vi "TLB Native Dynamic Events ver 0.04c.vi"() -> ()   [LabVIEW 2018]
uses:
  Labview Training Phase 2/Enum Controls/States for Action Engine.ctl
  Type def/TLB event states.ctl
  Type def/TLB MHL States.ctl
  <vilib>/Studica/Studica Toolkit/Background/I2C Channel.ctl
  <vilib>/Studica/Studica Toolkit/NavX/NavX.lvlib
  <vilib>/myRIO/Common/Instrument Driver Framework/myRIO v1.0/AI/typedefs/AI Channels Enum.ctl
  <vilib>/myRIO/Common/Instrument Driver Framework/myRIO v1.0/AI/typedefs/AI Channels List.ctl
  <vilib>/Studica/Studica Toolkit/Background/Mxp Selection.ctl
  <vilib>/ptbypt/NI_PtbyPt.lvlib
panel:
  out "Sharp IR Distance":dbl
  out "Sharp IR Distance 2":dbl
  out "CM":fxp<+,64,16>
  out "mean":dbl format="%0.2f"
  out "Waveform Chart 3":dbl(graph)
  out "NavX Info Out":T2
  out "LinearAcceleration":T3
  out "Displacement":T4
  out "YRPHfH":T5
  in  "xTargetSpeed":dbl
  in  "yTargetSpeed":dbl
  in  "wTargetSpeed":dbl
  out "Speed":T6
  in  "Reset Encoder 0":bool
  out "yDistance":dbl
  out "xDistance":dbl
  out "wDistance":dbl
  out "Action Queue Items":i32
  out "State Logic Queue Items":i32
  out "Action Queues items":string[](array[string])=["Hardware reset", "Software reset", ""]
  out "State logic":T7=enum."Task 2"
  out "Action State":string
  in  "Task Execution Mode":bool
  in  "Tasks Selector":string(combo)="Task 2"
  in  "Stop Queue":bool
  in  "Start Task":bool
  # "Test Programme written by Calvin Loke    Dated: 28 Aug 2019\nTest Programme revised by Dr Alex See   Dated 30 Aug 2019\n\nProgramme version:   TLB Native Dynamic Events ver 0.04b.vi"
  # "System Health Status Update"
  # "Sequence of Actions"
  # "Continuous (Repeated)"
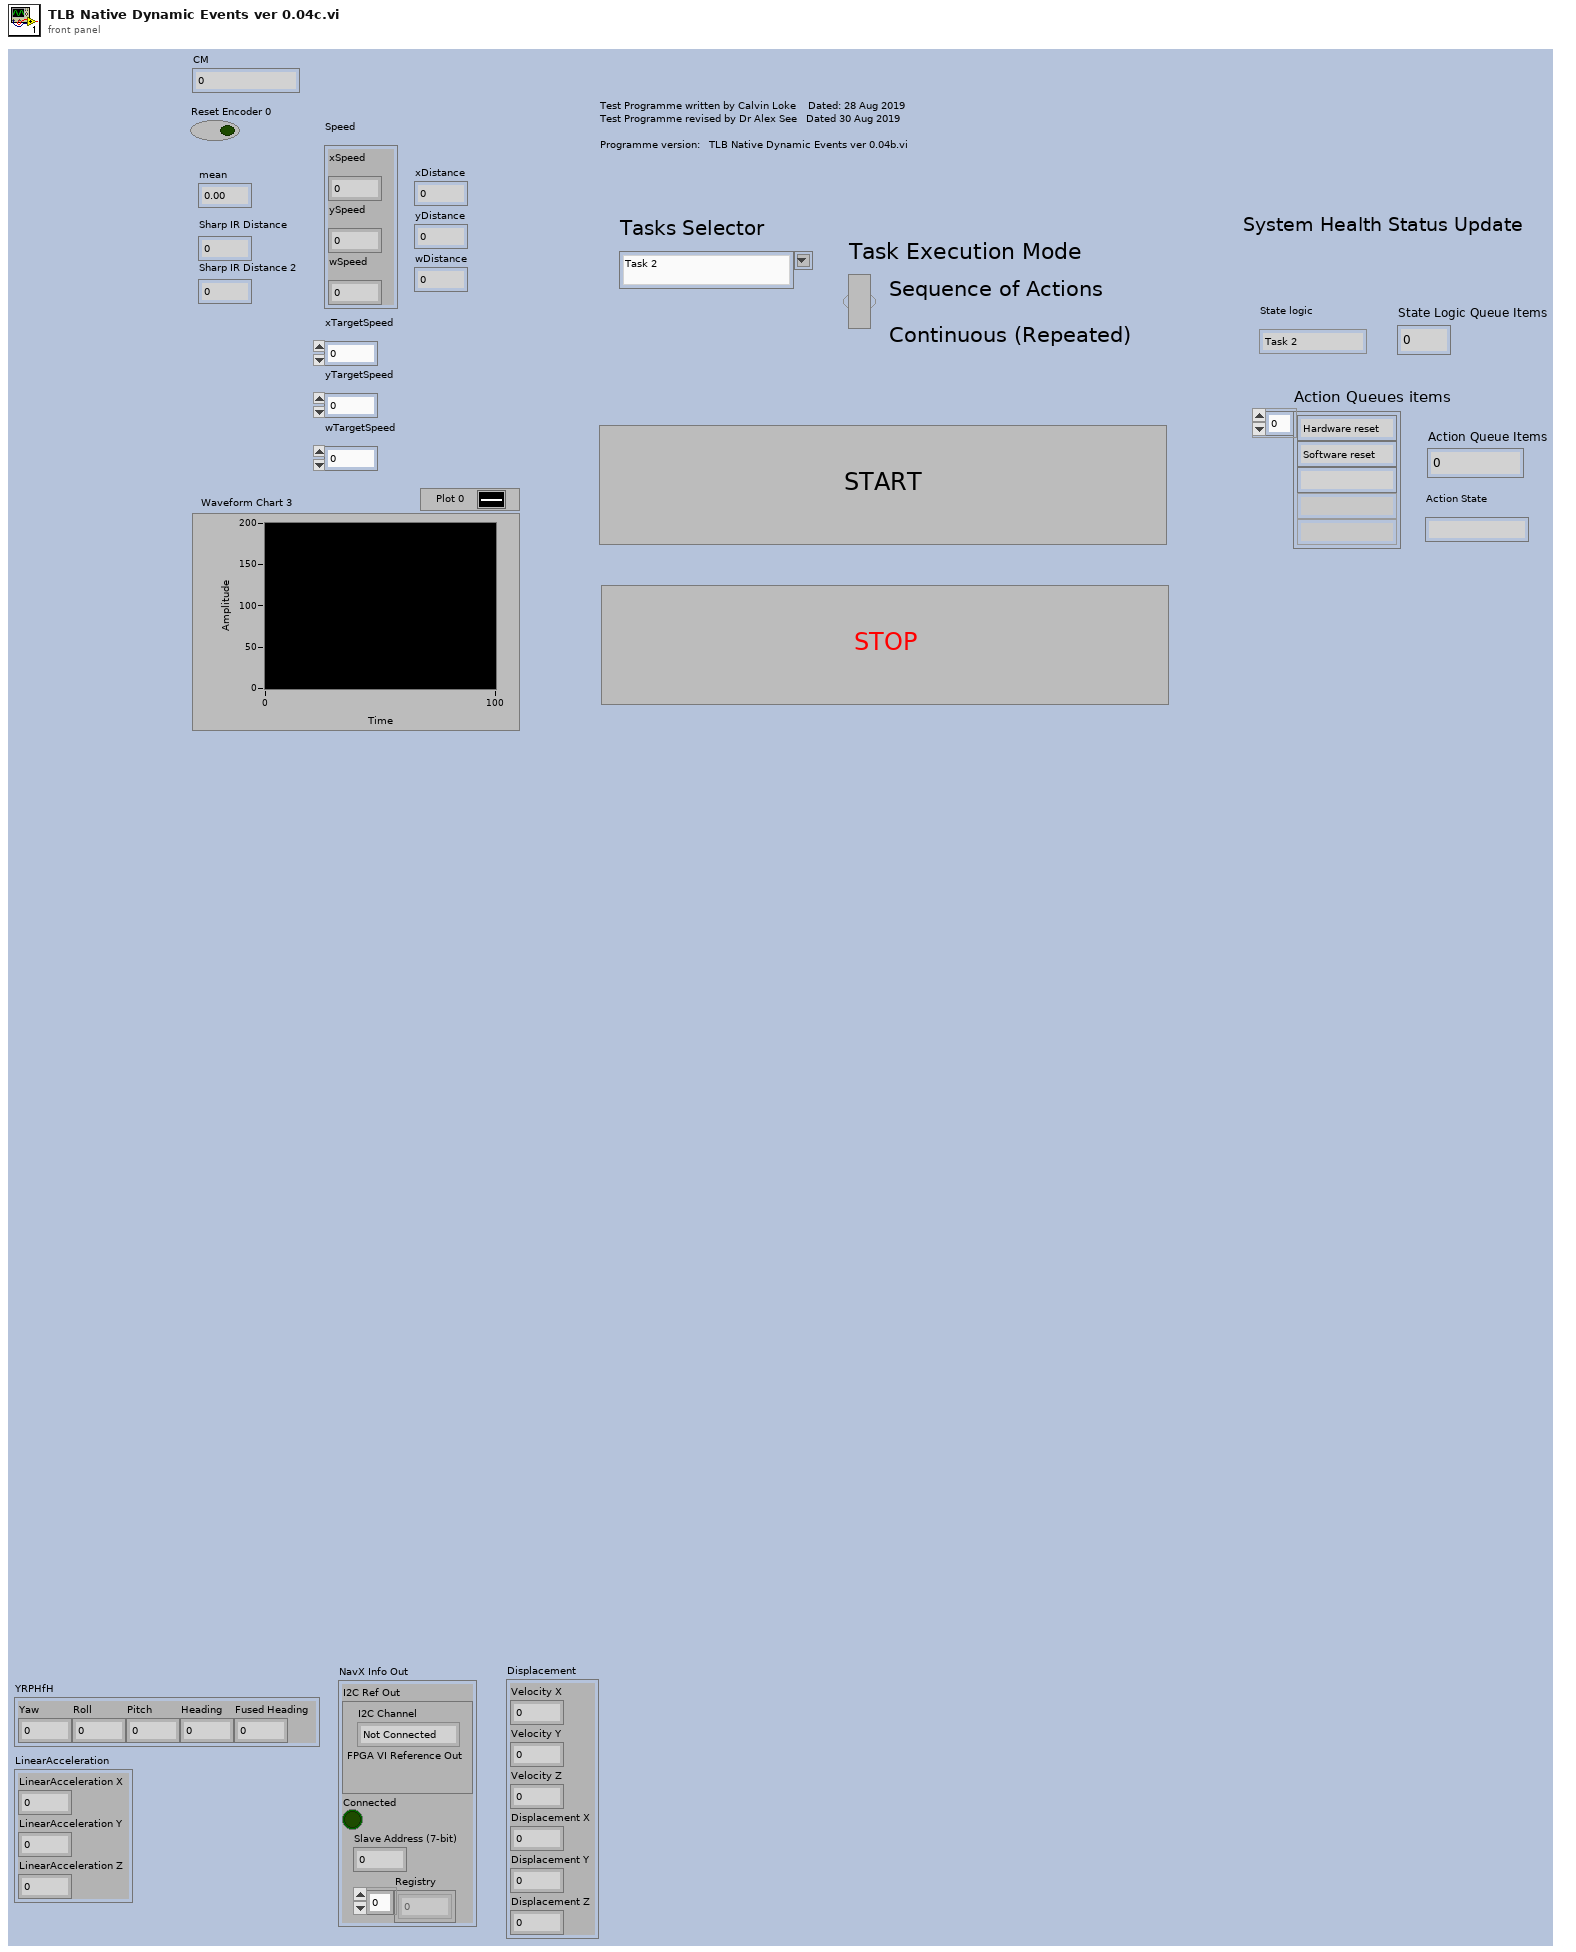
[diagram p1: front panel]
types:
  T1 = typedef "I2C Channel.ctl" = enum16{"Not Connected", "A", "B"}
  T2 = cluster{"I2C Ref Out":cluster{"I2C Channel":T1, "FPGA VI Reference Out":refnum<k20>}, "Connected":bool, "Slave Address (7-bit)":u8, "Registry":u8[]}
  T3 = cluster{"LinearAcceleration X":dbl, "LinearAcceleration Y":dbl, "LinearAcceleration Z":dbl}
  T4 = cluster{"Velocity X":dbl, "Velocity Y":dbl, "Velocity Z":dbl, "Displacement X":dbl, "Displacement Y":dbl, "Displacement Z":dbl}
  T5 = cluster{"Yaw":dbl, "Roll":dbl, "Pitch":dbl, "Heading":dbl, "Fused Heading":dbl}
  T6 = cluster{"xSpeed":dbl, "ySpeed":dbl, "wSpeed":dbl}
  T7 = typedef "TLB MHL States.ctl" = enum16{"None", "Startup", "Idle", "Processing", "Shutdown", "Reset", "Task 1", "Task 2", "Task 3", "Task 4", "Task 4a", "Task 4b", "Task 4c", "Task 4d", "Task 4e", "Task 4f", "Task 4g", "Task 4h", "Acquire image", "Wall follow mode", "Drive Straight"}
  T8 = typedef "States for Action Engine.ctl" = enum16{"Initialize", "Write", "Read"}
  T9 = typedef "TLB event states.ctl" = enum16{"Start Sequence", "Exit", "Start Task 1", "Start Task 2", "Start Task 3", "Start Task 4", "Camera vision", "Wall follow mode", "Idle", "Start Drive Straight"}
  T10 = typedef "Mxp Selection.ctl" = enum16{"MXP A", "MXP B"}
  T11 = typedef "TLB event states.ctl" = enum16{"Start Sequence", "Exit", "Task 1", "Task 2", "Idle"}
  T12 = typedef "AI Channels List.ctl" = T13[]
  T13 = typedef "AI Channels Enum.ctl" = enum16{"Not Connected", "AudioIn/Left", "AudioIn/Right", "C/AI0", "C/AI1", "A/AI0", "A/AI1", "A/AI2", "A/AI3", "A/AI4", "A/AI5", "A/AI6", "A/AI7", "B/AI0", "B/AI1", "B/AI2", "B/AI3", "B/AI4", "B/AI5", "B/AI6", "B/AI7", "AI/AI0", "AI/AI1", "AI/AI2", "AI/AI3", "A/AI0 (DIFF)", "A/AI1 (DIFF)", "A/AI2 (DIFF)", "A/AI3 (DIFF)", "B/AI0 (DIFF)", "B/AI1 (DIFF)", "B/AI2 (DIFF)", "B/AI3 (DIFF)"}
  T14 = cluster{"xDistance":dbl, "yDistance":dbl, "wDistance":dbl}
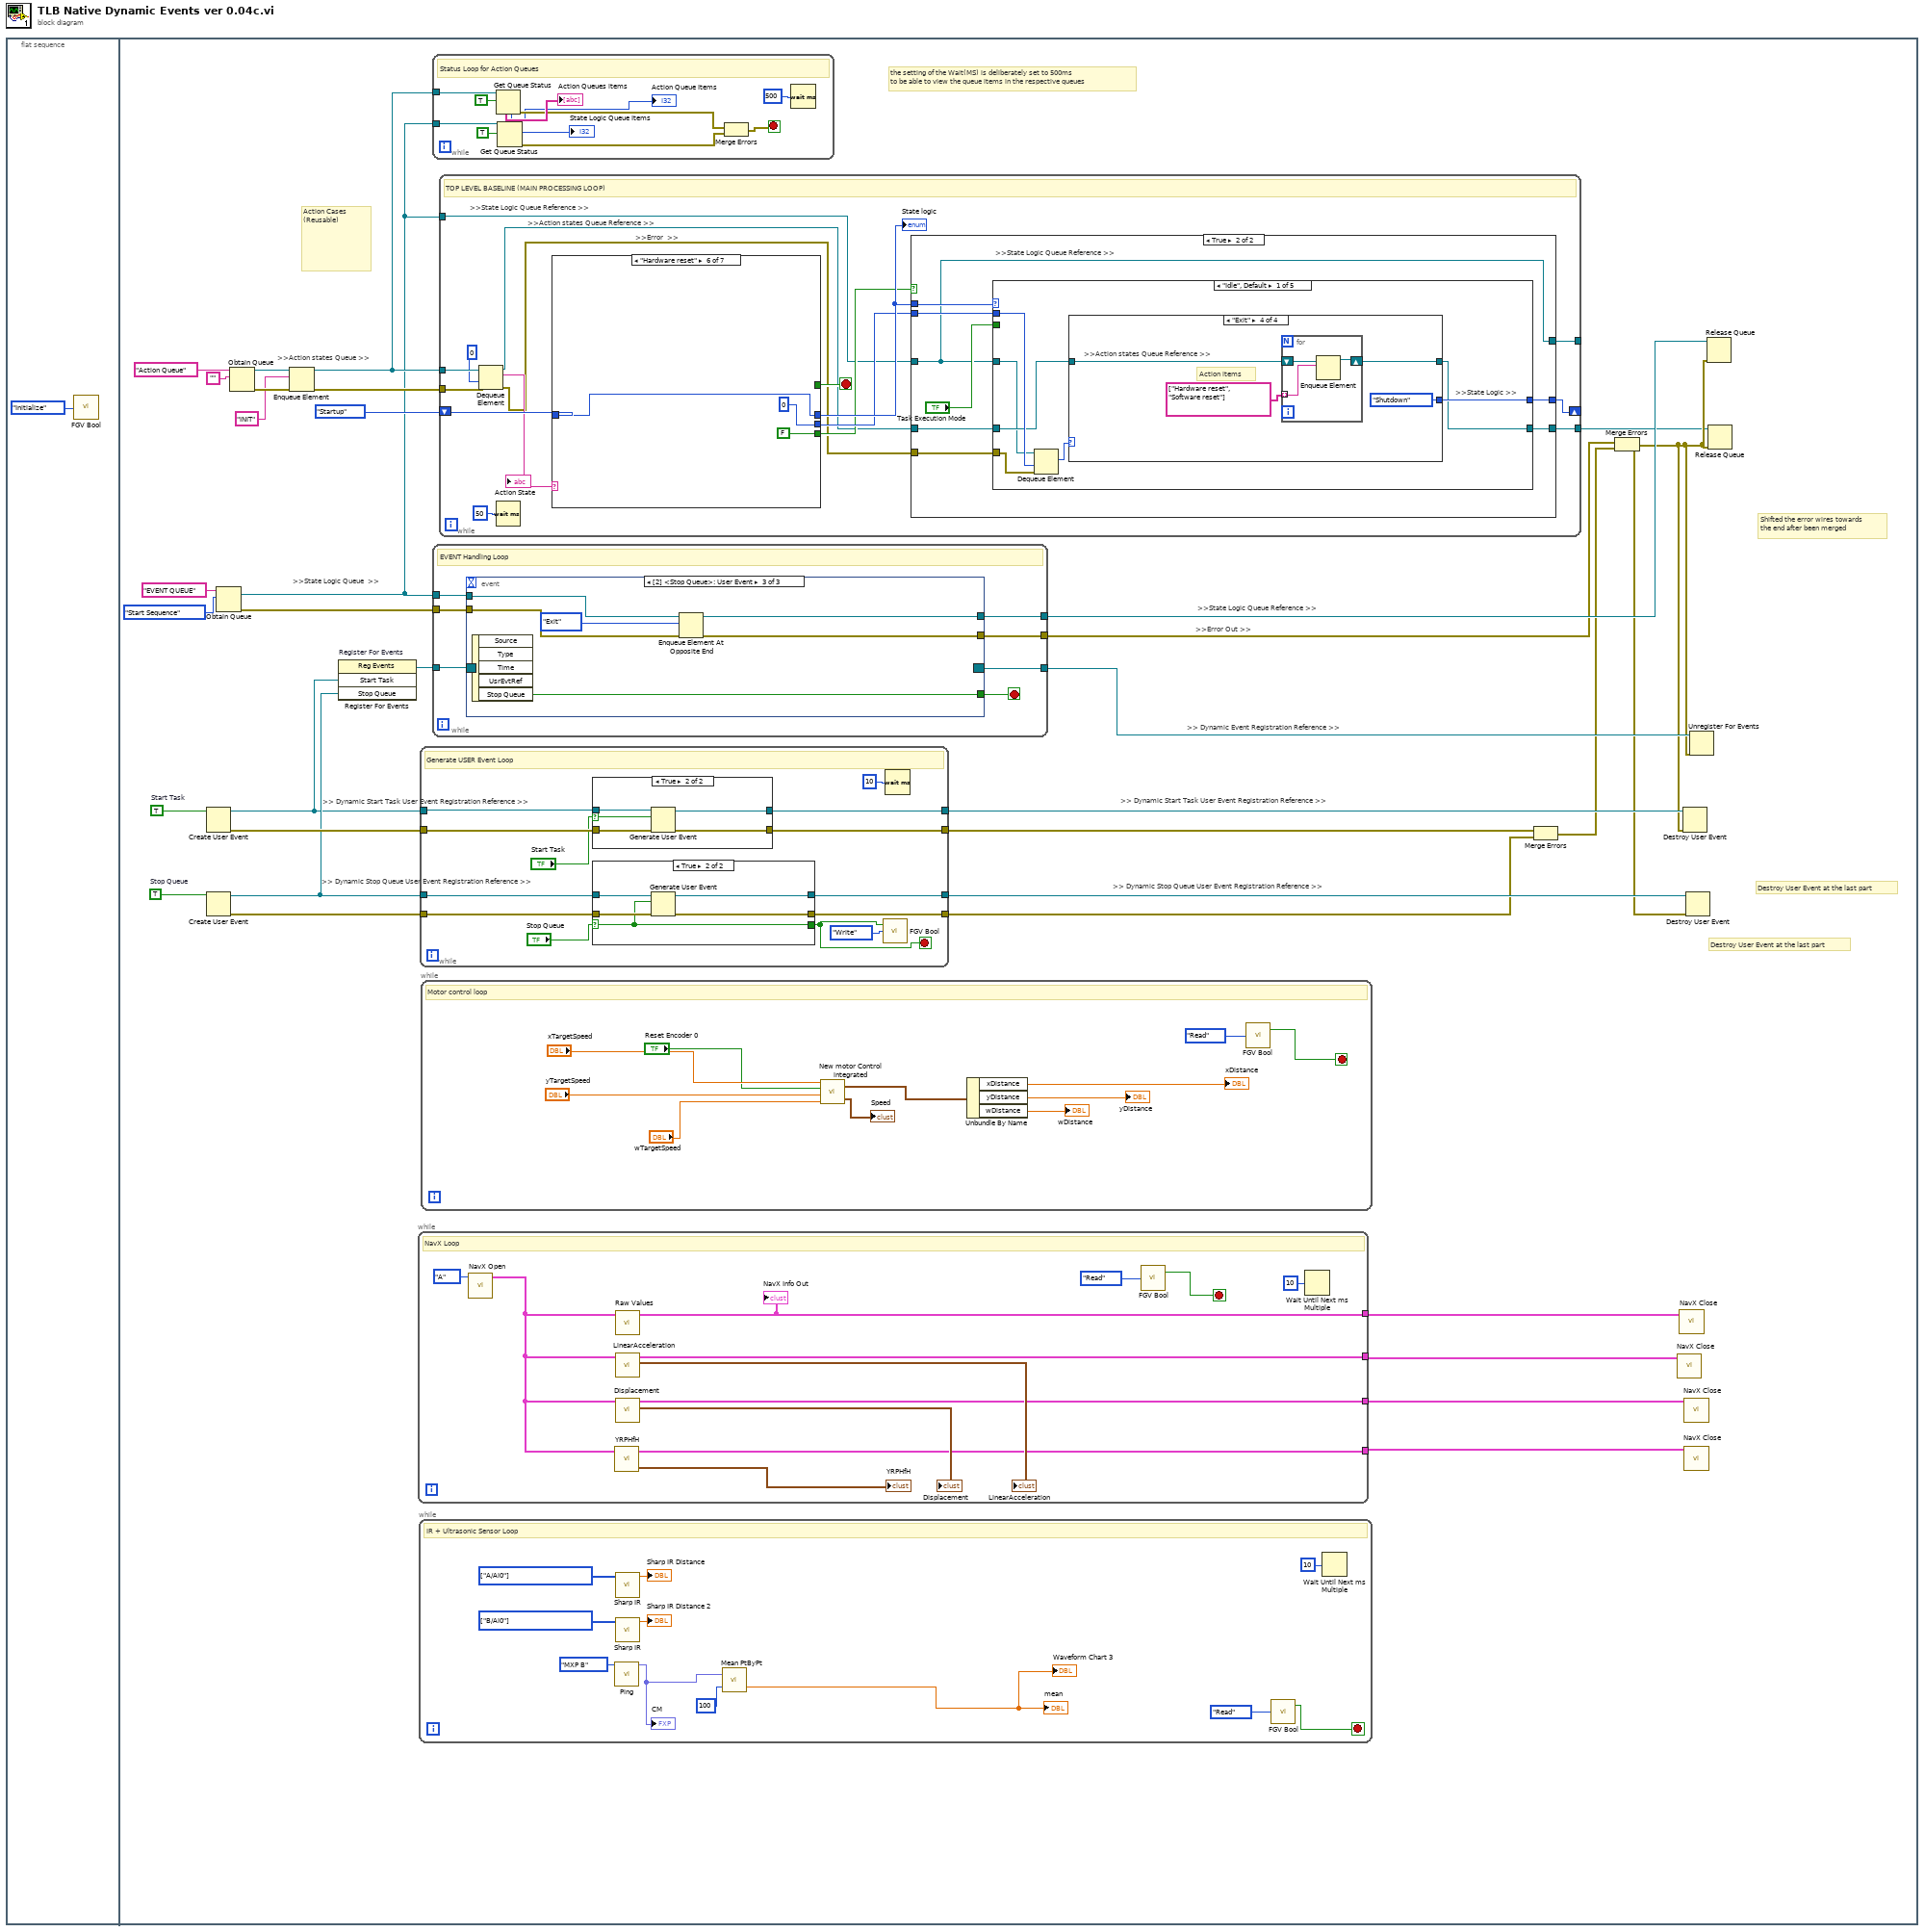
[diagram p0: block diagram]
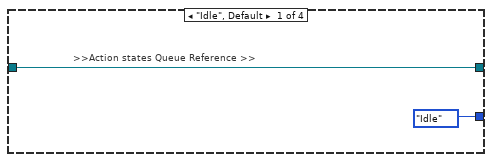
[diagram p3: hidden frame]
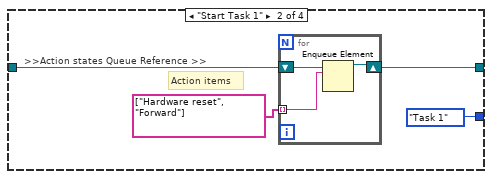
[diagram p4: hidden frame]
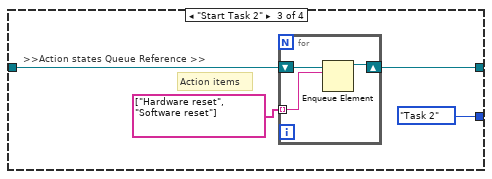
[diagram p5: hidden frame]
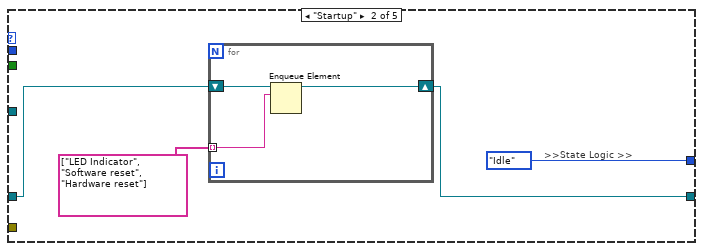
[diagram p6: hidden frame]
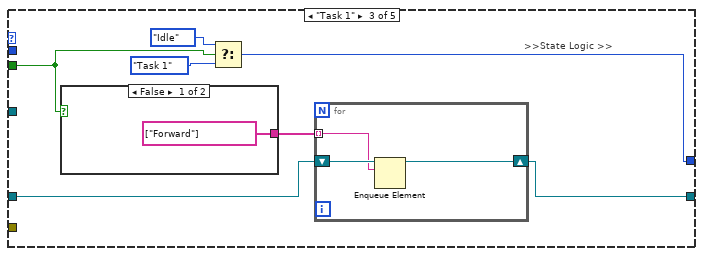
[diagram p7: hidden frame]
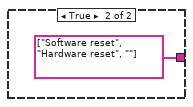
[diagram p8: hidden frame]
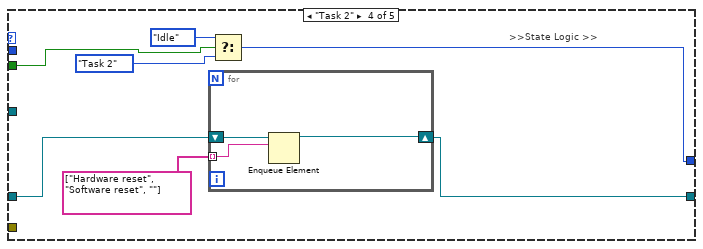
[diagram p9: hidden frame]
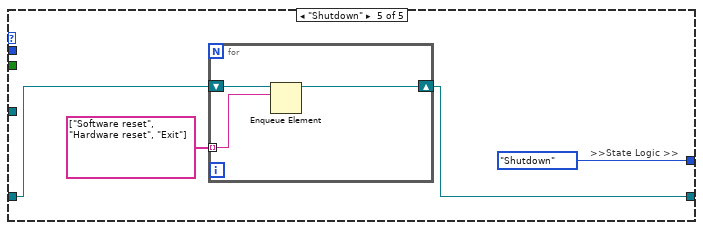
[diagram p10: hidden frame]
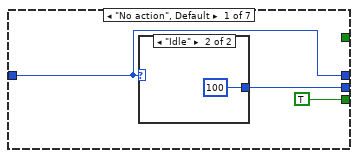
[diagram p11: hidden frame]
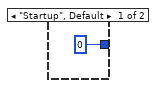
[diagram p12: hidden frame]
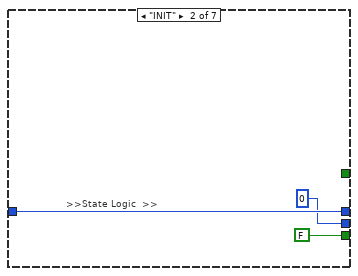
[diagram p13: hidden frame]
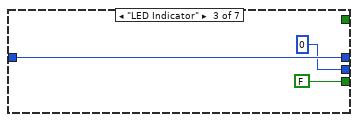
[diagram p14: hidden frame]
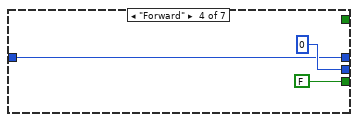
[diagram p15: hidden frame]
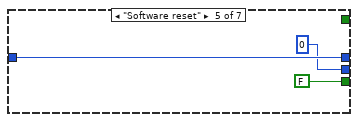
[diagram p16: hidden frame]
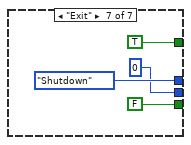
[diagram p17: hidden frame]
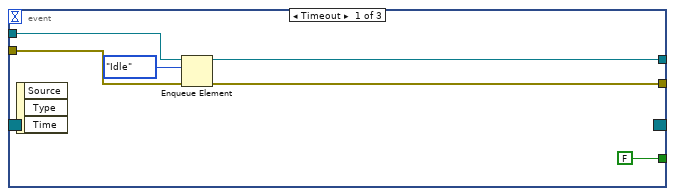
[diagram p18: hidden frame]
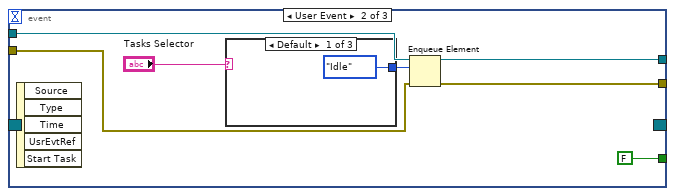
[diagram p19: hidden frame]
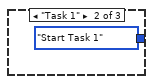
[diagram p20: hidden frame]
diagram:
  n1 = flat-sequence {
    frame #0 {
      n2 = call "FGV Bool.vi"("Init/Read/Write State"=States_for_Action_Engine."Initialize") -> ()  [unwired: 2 in, 2 out]
    }
    frame #1 {
      w34 = TRUE  # Stop Queue
      w33 = TRUE  # Start Task
      # "the setting of the Wait(MS) is deliberately set to 500ms\nto be able to view the queue items in the respective queues"
      # "Action Cases\n(Reusable)"
      # ">>Error Out >>"
      # ">> Dynamic Stop Queue User Event Registration Reference >>"
      # ">> Dynamic Start Task User Event Registration Reference >>"
      # ">> Dynamic Stop Queue User Event Registration Reference >>"
      # ">> Dynamic Start Task User Event Registration Reference >>"
      # ">> Dynamic Event Registration Reference >>"
      # ">>Action states Queue >>"
      # ">>State Logic Queue  >>"
      # ">>State Logic Queue Reference >>"
      # "Destroy User Event at the last part"
      # "Destroy User Event at the last part"
      # "Shifted the error wires towards\nthe end after been merged"
      n3 = Create User Event(user event datatype=w33) -> (user event=w25:refnum<user-event>, error out=w30:errorcluster)  [unwired: 1 in]
      n4 = Create User Event(user event datatype=w34) -> (user event=w26:refnum<user-event>, error out=w29:errorcluster)  [unwired: 1 in]
      n5 = Obtain Queue(name (unnamed)="EVENT QUEUE", element data type=TLB_event_states."Start Sequence" ("Enum")) -> (queue out=w9:refnum<queue>, error out=w15:errorcluster)  [unwired: 3 in, 1 out]
      n6 = Obtain Queue(name (unnamed)="Action Queue", element data type="") -> (queue out=w18:refnum<queue>, error out=w14:errorcluster)  [unwired: 3 in, 1 out]
      n7 = Enqueue Element(queue=w18, element="INIT", error in (no error)=w14) -> (queue out=w10:refnum<queue>, error out=w13:errorcluster)  [unwired: 1 in, 1 out]
      n8 = register-events "Register For Events"(w25, w26) -> (reference out=w24:refnum<event-registration>)  [unwired: 2 in, 1 out]
      n9 = while {
        tunnel: [w54] -> w5
        tunnel: [w50] -> w4
        tunnel: [w49] -> w2
        tunnel: [w48] -> w3
        stop <- w56 stop-if-true
        # "NavX Loop"
        n10 = call <vilib>:"NavX Open.vi"("I2C Channel"=I2C_Channel."A") -> ("NavX Info"=w46:T2)  [unwired: 9 in, 1 out]
        n11 = call <vilib>:"YRPHfH.vi"("NavX Info In"=w46) -> ("YRPHfH"=→"YRPHfH":T5, "NavX Info Out"=w49:T2)  [unwired: 3 in]
        n12 = call <vilib>:"Raw Values.vi"("NavX Info In"=w46) -> ("NavX Info Out"=w54:T2)  [unwired: 8 in, 1 out]
        "NavX Info Out" <- w54
        n13 = call <vilib>:"LinearAcceleration.vi"("NavX Info In"=w46) -> ("LinearAcceleration"=→"LinearAcceleration":T3, "NavX Info Out"=w50:T2)  [unwired: 9 in]
        n14 = call <vilib>:"Displacement.vi"("NavX Info In"=w46) -> ("Displacement"=→"Displacement":T4, "NavX Info Out"=w48:T2)  [unwired: 9 in]
        n15 = call "FGV Bool.vi"("Init/Read/Write State"=States_for_Action_Engine."Read") -> ("Output node"=w56:bool)  [unwired: 2 in, 1 out]
        n16 = Wait Until Next ms Multiple(millisecond multiple=u32 10) -> ()  [unwired: 1 out]
      }
      n17 = while {
        stop <- w39 stop-if-true
        w44 = T12 [enum."B/AI0"] items=["Not Connected", "AudioIn/Left", "AudioIn/Right", "C/AI0", "C/AI1", "A/AI0", "A/AI1", "A/AI2", "A/AI3", "A/AI4", "A/AI5", "A/AI6", "A/AI7", "B/AI0", "B/AI1", "B/AI2", "B/AI3", "B/AI4", "B/AI5", "B/AI6", "B/AI7", "AI/AI0", "AI/AI1", "AI/AI2", "AI/AI3", "A/AI0 (DIFF)", "A/AI1 (DIFF)", "A/AI2 (DIFF)", "A/AI3 (DIFF)", "B/AI0 (DIFF)", "B/AI1 (DIFF)", "B/AI2 (DIFF)", "B/AI3 (DIFF)"] ("AI Channel")
        w45 = T12 [enum."A/AI0"] items=["Not Connected", "AudioIn/Left", "AudioIn/Right", "C/AI0", "C/AI1", "A/AI0", "A/AI1", "A/AI2", "A/AI3", "A/AI4", "A/AI5", "A/AI6", "A/AI7", "B/AI0", "B/AI1", "B/AI2", "B/AI3", "B/AI4", "B/AI5", "B/AI6", "B/AI7", "AI/AI0", "AI/AI1", "AI/AI2", "AI/AI3", "A/AI0 (DIFF)", "A/AI1 (DIFF)", "A/AI2 (DIFF)", "A/AI3 (DIFF)", "B/AI0 (DIFF)", "B/AI1 (DIFF)", "B/AI2 (DIFF)", "B/AI3 (DIFF)"] ("AI Channel")
        # "IR + Ultrasonic Sensor Loop"
        n18 = call <vilib>:"Ping.vi"("Mxp Side"=Mxp_Selection."MXP B") -> ("CM"=w35:fxp<+,64,16>)  [unwired: 8 in, 2 out]
        "CM" <- w35
        n19 = call <vilib>:"Sharp IR.vi"("AI Channel"=w45) -> ("Sharp IR Distance"=→"Sharp IR Distance":dbl)  [unwired: 8 in, 2 out]
        n20 = call <vilib>:"Sharp IR.vi"("AI Channel"=w44) -> ("Sharp IR Distance"=→"Sharp IR Distance 2":dbl)  [unwired: 8 in, 2 out]
        n21 = call <vilib>:"Mean PtByPt.vi"("x"=w35, "sample length"=100) -> ("mean"=→"mean" →"Waveform Chart 3":dbl)  [unwired: 2 in, 1 out]
        n22 = call "FGV Bool.vi"("Init/Read/Write State"=States_for_Action_Engine."Read") -> ("Output node"=w39:bool)  [unwired: 2 in, 1 out]
        n23 = Wait Until Next ms Multiple(millisecond multiple=u32 10) -> ()  [unwired: 1 out]
      }
      n24 = while {
        tunnel: w25 -> [w237]
        tunnel: w26 -> [w236]
        tunnel: [w235] -> w32
        tunnel: [w234] -> w31
        tunnel: w30 -> [w233]
        tunnel: [w232] -> w28
        tunnel: w29 -> [w231]
        tunnel: [w230] -> w27
        stop <- w226 stop-if-true
        # "Generate USER Event Loop"
        n25 = case shown="True" "Start Task" {
          selector: "Start Task" -> [_ w249]
          tunnel: w237 -> [w248 w253]
          tunnel: [w248 w252] -> w234
          tunnel: w233 -> [w247 w251]
          tunnel: [w247 w250] -> w232
          frame False {
          }
          frame True {
            n26 = Generate User Event(user event=w253, event data cluster=w249, error in=w251) -> (user event out=w252:refnum<user-event>, error out=w250:errorcluster)  [unwired: 1 in]
          }
        }
        n27 = case shown="True" "Stop Queue" {
          selector: "Stop Queue" -> [_ w242]
          tunnel: w236 -> [w241 w246]
          tunnel: [w241 w245] -> w235
          tunnel: w231 -> [w240 w244]
          tunnel: [w240 w243] -> w230
          tunnel: [FALSE w242] -> w226
          frame False {
          }
          frame True {
            n28 = Generate User Event(user event=w246, event data cluster=w242, error in=w244) -> (user event out=w245:refnum<user-event>, error out=w243:errorcluster)  [unwired: 1 in]
          }
        }
        n29 = call "FGV Bool.vi"("Init/Read/Write State"=States_for_Action_Engine."Write", "Input Node"=w226) -> ()  [unwired: 1 in, 2 out]
        n30 = Wait (ms)(milliseconds to wait=u32 10) -> ()  [unwired: 1 out]
      }
      n31 = while {
        stop <- w67 stop-if-true
        # "Motor control loop"
        n32 = call "New motor Control integrated.vi"("wTargetSpeed"="wTargetSpeed", "yTargetSpeed"="yTargetSpeed", "xTargetSpeed"="Reset Encoder 0", "Reset Encoders"="xTargetSpeed") -> ("Speed"=→"Speed":T6, "Distance"=w61:T14)
        n33 = Unbundle By Name(w61) -> ("xDistance"=→"xDistance":dbl, "yDistance"=→"yDistance":dbl, "wDistance"=→"wDistance":dbl)
        n34 = call "FGV Bool.vi"("Init/Read/Write State"=States_for_Action_Engine."Read") -> ("Output node"=w67:bool)  [unwired: 2 in, 1 out]
      }
      n35 = while {
        tunnel: w10 -> [w77]
        tunnel: w9 -> [w74]
        stop <- w71 stop-if-true
        # "Status Loop for Action Queues"
        n36 = Get Queue Status(queue=w77, return elements? (F)=TRUE) -> (error out=w73:errorcluster, # elements in queue=→"Action Queue Items":i32, elements=→"Action Queues items":string[])  [unwired: 1 in, 5 out]
        n37 = Get Queue Status(queue=w74, return elements? (F)=TRUE) -> (# pending remove=→"State Logic Queue Items":i32, error out=w72:errorcluster)  [unwired: 1 in, 6 out]
        n38 = Merge Errors(w73, w72) -> (w71:errorcluster)
        n39 = Wait (ms)(milliseconds to wait=u32 500) -> ()  [unwired: 1 out]
      }
      n40 = while {
        tunnel: w24 -> [w203]
        tunnel: [w202] -> w23
        tunnel: w9 -> [w200]
        tunnel: [w199] -> w22
        tunnel: w15 -> [w198]
        tunnel: [w197] -> w12
        stop <- w201 stop-if-true
        # "EVENT Handling Loop"
        n41 = event shown="[2] <Stop Queue>: User Event" {
          selector: w203 -> [_ _ _]
          dyn-events: [_ _ _] -> w202
          timeout: _ -> [_ _ _]
          tunnel: [FALSE FALSE w225] -> w201
          tunnel: w200 -> [w208 w215 w223]
          tunnel: [w207 w214 w224] -> w199
          tunnel: w198 -> [w205 w211 w221]
          tunnel: [w204 w210 w220] -> w197
          event Timeout {
            n42 = event-data() -> ()  [unwired: 1 in, 3 out]
            n43 = Enqueue Element(queue=w208, element=TLB_event_states."Idle" ("Enum"), error in (no error)=w205) -> (queue out=w207:refnum<queue>, error out=w204:errorcluster)  [unwired: 1 in, 1 out]
          }
          event User Event {
            n44 = event-data() -> ()  [unwired: 1 in, 5 out]
            n45 = case shown="Default" "Tasks Selector" {
              tunnel: [TLB_event_states."Idle" ("Enum") TLB_event_states."Start Task 1" ("Enum") TLB_event_states."Task 2" ("Enum")] -> w212
              frame Default {
              }
              frame "Task 1" {
              }
              frame "Task 2" {
              }
            }
            n46 = Enqueue Element(queue=w215, element=w212, error in (no error)=w211) -> (queue out=w214:refnum<queue>, error out=w210:errorcluster)  [unwired: 1 in, 1 out]
          }
          event User Event {
            n47 = event-data() -> ("Stop Queue"=w225:bool)  [unwired: 1 in, 4 out]
            n48 = Enqueue Element At Opposite End(queue=w223, element=TLB_event_states."Exit" ("Enum"), error in (no error)=w221) -> (queue out=w224:refnum<queue>, error out=w220:errorcluster)  [unwired: 1 in, 1 out]
          }
        }
      }
      n49 = while {
        tunnel: w9 -> [w82]
        shift-right: [w87] -> _
        shift-left: TLB_MHL_States."Startup" ("Enum") -> [w94]
        tunnel: w10 -> [w92]
        tunnel: w13 -> [w90]
        tunnel: [w89] -> _
        tunnel: [w88] -> w7
        stop <- w85 stop-if-true
        # ">>Error  >>"
        # ">>Action states Queue Reference >>"
        # ">>State Logic Queue Reference >>"
        # "TOP LEVEL BASELINE (MAIN PROCESSING LOOP)"
        n50 = Dequeue Element(queue=w92, timeout in ms (-1)=0, error in (no error)=w90) -> (queue out=w81:refnum<queue>, element=w91:string, error out=w80:errorcluster)  [unwired: 1 out]
        "Action State" <- w91
        n51 = Wait (ms)(milliseconds to wait=u32 50) -> ()  [unwired: 1 out]
        n52 = case shown="\"Hardware reset\"" w91 {
          tunnel: [w175 w180 w183 w185 w189 w192 TLB_MHL_States."Shutdown" ("Enum")] -> w93
          tunnel: w94 -> [w175 w180 w183 w185 w189 w192 _]
          tunnel: [w174 0 0 0 0 0 0] -> w86
          tunnel: [_ _ _ _ _ _ TRUE] -> w85
          tunnel: [TRUE FALSE FALSE FALSE FALSE FALSE FALSE] -> w84
          frame "No action", Default {
            n53 = case shown="\"Idle\"" w175 {
              tunnel: [0 100] -> w174
              frame "Startup", Default {
              }
              frame "Idle" {
              }
            }
          }
          frame "INIT" {
            # ">>State Logic  >>"
          }
          frame "LED Indicator" {
          }
          frame "Forward" {
          }
          frame "Software reset" {
          }
          frame "Hardware reset" {
          }
          frame "Exit" {
          }
        }
        "State logic" <- w93
        n54 = case shown="True" w84 {
          tunnel: w93 -> [w97 w106]
          tunnel: w82 -> [w98 w99]
          tunnel: w81 -> [w96 w105]
          tunnel: [w98 w99] -> w89
          tunnel: [w96 w104] -> w88
          tunnel: [w97 w103] -> w87
          tunnel: w80 -> [_ w102]
          tunnel: w86 -> [_ w101]
          frame False {
          }
          frame True {
            # ">>State Logic Queue Reference >>"
            n55 = case shown="\"Idle\", Default" w106 {
              tunnel: w99 -> [w107 _ _ _ _]
              tunnel: w105 -> [w109 w138 w145 w157 w167]
              tunnel: [w108 w137 w144 w158 w166] -> w104
              tunnel: [w112 TLB_MHL_States."Idle" ("Enum") w148 w160 TLB_MHL_States."Shutdown" ("Enum")] -> w103
              tunnel: w102 -> [w110 _ _ _ _]
              tunnel: w101 -> [w111 _ _ _ _]
              tunnel: "Task Execution Mode" -> [_ _ w147 w156 _]
              frame "Idle", Default {
                # ">>State Logic >>"
                n56 = Dequeue Element(queue=w107, timeout in ms (-1)=w111, error in (no error)=w110) -> (element=w113:T9)  [unwired: 3 out]
                n57 = case shown="\"Exit\"" w113 {
                  tunnel: [TLB_MHL_States."Idle" ("Enum") TLB_MHL_States."Task 1" ("Enum") TLB_MHL_States."Task 2" ("Enum") TLB_MHL_States."Shutdown" ("Enum")] -> w112
                  tunnel: [w114 w118 w123 w130] -> w108
                  tunnel: w109 -> [w114 w116 w124 w131]
                  frame "Idle", Default {
                    # ">>Action states Queue Reference >>"
                  }
                  frame "Start Task 1" {
                    # ">>Action states Queue Reference >>"
                    # "Action items"
                    n58 = for {
                      shift-right: [w122] -> w118
                      shift-left: w116 -> [w121]
                      tunnel: string[] ["Hardware reset", "Forward"] -> [w120] mode=indexing
                      n59 = Enqueue Element(queue=w121, element=w120) -> (queue out=w122:refnum<queue>)  [unwired: 2 in, 2 out]
                    }
                  }
                  frame "Start Task 2" {
                    # ">>Action states Queue Reference >>"
                    # "Action items"
                    n60 = for {
                      shift-right: [w129] -> w123
                      shift-left: w124 -> [w128]
                      tunnel: string[] ["Hardware reset", "Software reset"] -> [w127] mode=indexing
                      n61 = Enqueue Element(queue=w128, element=w127) -> (queue out=w129:refnum<queue>)  [unwired: 2 in, 2 out]
                    }
                  }
                  frame "Exit" {
                    # ">>Action states Queue Reference >>"
                    # "Action items"
                    n62 = for {
                      shift-right: [w136] -> w130
                      shift-left: w131 -> [w135]
                      tunnel: string[] ["Hardware reset", "Software reset"] -> [w134] mode=indexing
                      n63 = Enqueue Element(queue=w135, element=w134) -> (queue out=w136:refnum<queue>)  [unwired: 2 in, 2 out]
                    }
                  }
                }
              }
              frame "Startup" {
                # ">>State Logic >>"
                n64 = for {
                  shift-right: [w142] -> w137
                  shift-left: w138 -> [w143]
                  tunnel: string[] ["LED Indicator", "Software reset", "Hardware reset"] -> [w141] mode=indexing
                  n65 = Enqueue Element(queue=w143, element=w141) -> (queue out=w142:refnum<queue>)  [unwired: 2 in, 2 out]
                }
              }
              frame "Task 1" {
                # ">>State Logic >>"
                n66 = case shown="False" w147 {
                  tunnel: [string[] ["Forward"] string[] ["Software reset", "Hardware reset", ""]] -> w146
                  frame False {
                  }
                  frame True {
                  }
                }
                n67 = Select(t=TLB_MHL_States."Idle" ("Enum"), s=w147, f=TLB_MHL_States."Task 1" ("Enum")) -> (s? t:f=w148:T7)
                n68 = for {
                  shift-right: [w154] -> w144
                  shift-left: w145 -> [w155]
                  tunnel: w146 -> [w153] mode=indexing
                  n69 = Enqueue Element(queue=w155, element=w153) -> (queue out=w154:refnum<queue>)  [unwired: 2 in, 2 out]
                }
              }
              frame "Task 2" {
                # ">>State Logic >>"
                n70 = for {
                  shift-right: [w164] -> w158
                  shift-left: w157 -> [w165]
                  tunnel: string[] ["Hardware reset", "Software reset", ""] -> [w163] mode=indexing
                  n71 = Enqueue Element(queue=w165, element=w163) -> (queue out=w164:refnum<queue>)  [unwired: 2 in, 2 out]
                }
                n72 = Select(t=TLB_MHL_States."Idle" ("Enum"), s=w156, f=TLB_MHL_States."Task 2" ("Enum")) -> (s? t:f=w160:T7)
              }
              frame "Shutdown" {
                # ">>State Logic >>"
                n73 = for {
                  shift-right: [w171] -> w166
                  shift-left: w167 -> [w172]
                  tunnel: string[] ["Software reset", "Hardware reset", "Exit"] -> [w170] mode=indexing
                  n74 = Enqueue Element(queue=w172, element=w170) -> (queue out=w171:refnum<queue>)  [unwired: 2 in, 2 out]
                }
              }
            }
          }
        }
      }
      n75 = Merge Errors "Merge Errors"(w28, w27) -> (w6:errorcluster)
      n76 = Merge Errors(w12, w6) -> (w8:errorcluster)
      n77 = call <vilib>:"NavX Close.vi"("NavX Info In"=w4) -> ()  [unwired: 10 in, 1 out]
      n78 = call <vilib>:"NavX Close.vi"("NavX Info In"=w5) -> ()  [unwired: 10 in, 1 out]
      n79 = Destroy User Event(user event=w31, error in=w8) -> ()  [unwired: 1 out]
      n80 = call <vilib>:"NavX Close.vi"("NavX Info In"=w3) -> ()  [unwired: 10 in, 1 out]
      n81 = call <vilib>:"NavX Close.vi"("NavX Info In"=w2) -> ()  [unwired: 10 in, 1 out]
      n82 = Destroy User Event(user event=w32, error in=w8) -> ()  [unwired: 1 out]
      n83 = Unregister For Events(event registration refnum=w23, error in=w8) -> ()  [unwired: 1 out]
      n84 = Release Queue(queue=w22, error in (no error)=w8) -> ()  [unwired: 1 in, 3 out]
      n85 = Release Queue(queue=w7, error in (no error)=w8) -> ()  [unwired: 1 in, 3 out]
    }
  }
